vi "Get Control Refs and Names.vi"(11 "Controls[]":refnum<vi>[](array[refnum])) -> (2 "Ctrl Labels":string[](array[string]), 3 "Ctrl Refs":refnum<vi>[](array[refnum]))   [LabVIEW 2018, in "EMS User Interface Actor.lvlib" / "EMS User Interface.lvclass"]
uses:
  EMS User Interface.lvclass
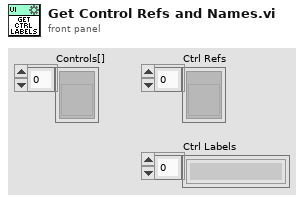
[diagram p1: front panel]
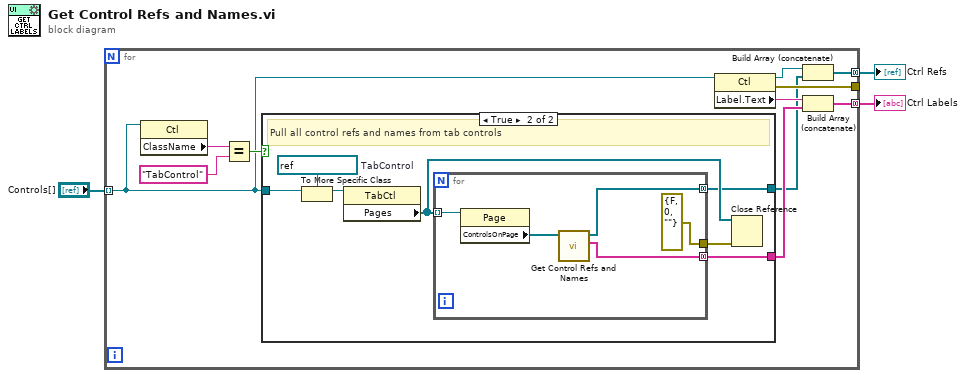
[diagram p0: block diagram]
diagram:
  n1 = for {
    tunnel: "Controls[]" -> [w11] mode=indexing
    tunnel: [w7] -> w2 mode=concatenating
    tunnel: [w14] -> _
    tunnel: [w4] -> w3 mode=concatenating
    n2 = property class="Ctl"(reference=w11) -> ("ClassName"=w10:string)  [unwired: 1 in, 2 out]
    n3 = Equal?(x=w10, y="TabControl") -> (x = y?=w12:bool)
    n4 = case shown="True" w12 {
      tunnel: w11 -> [_ w21]
      tunnel: [_ w18] -> w9
      tunnel: [_ w16] -> w5
      frame False {
      }
      frame True {
        w20 = refnum<vi> refnum  # TabControl
        # "Pull all control refs and names from tab controls"
        n5 = To More Specific Class(target class=w20, reference=w21) -> (specific class reference=w19:refnum<vi>)  [unwired: 1 in, 1 out]
        n6 = property class="TabCtl"(reference=w19) -> ("Pages"=w17:refnum<vi>[])  [unwired: 1 in, 2 out]
        n7 = for {
          tunnel: w17 -> [w26] mode=indexing
          tunnel: [w23] -> w18 mode=concatenating
          tunnel: [w24] -> w16 mode=concatenating
          tunnel: [errorcluster {"status"=FALSE, "code"=0, "source"=""} ("error in (no error)")] -> w15
          n8 = property class="Page"(reference=w26) -> ("ControlsOnPage"=w25:refnum<vi>[])  [unwired: 1 in, 2 out]
          n9 = call "Get Control Refs and Names.vi"("Controls[]"=w25) -> ("Ctrl Labels"=w23:string[], "Ctrl Refs"=w24:refnum<vi>[])  [unwired: 9 in]
        }
        n10 = Close Reference(reference=w17, error in (no error)=w15) -> ()  [unwired: 1 out]
      }
    }
    n11 = property class="Ctl"(reference=w11) -> (reference out=w6:refnum<vi>, error out=w14:errorcluster, "Label.Text"=w8:string)  [unwired: 1 in]
    n12 = Build Array (concatenate)(w6, w5) -> (w4:refnum<vi>[])
    n13 = Build Array (concatenate)(w8, w9) -> (w7:string[])
  }
  "Ctrl Refs" <- w3
  "Ctrl Labels" <- w2
